vi "Position FLight Mode Enum.vi"(8 "error in (no error)":errorcluster, 10 "TabCtl Refnum":refnum<vi>, 11 "Enum Refnum":refnum<vi>) -> (0 "error out":errorcluster)   [LabVIEW 2014]
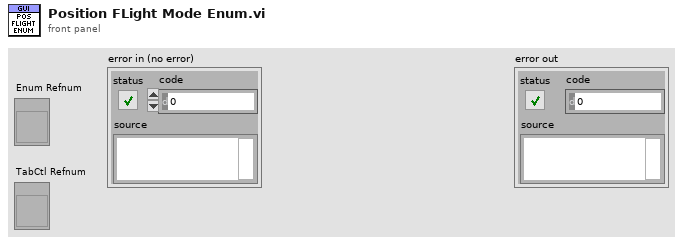
[diagram p1: front panel]
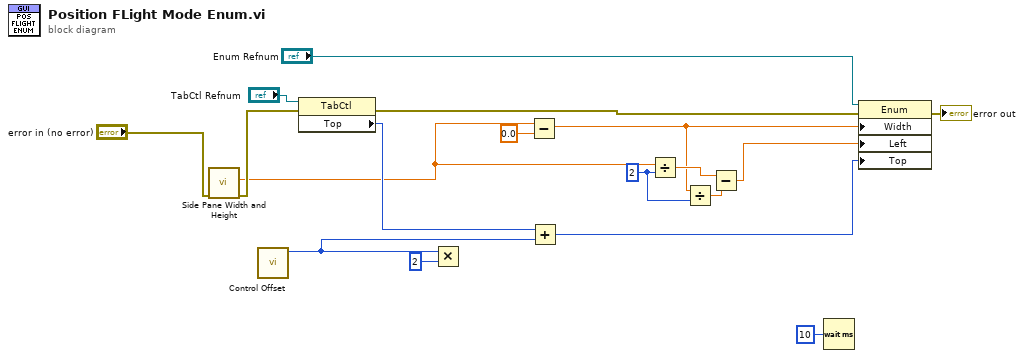
[diagram p0: block diagram]
diagram:
  w10 = u32 2 ("y")
  n1 = call "Side Pane Width and Height.vi"("error in (no error)"="error in (no error)") -> ("error out"=w3:errorcluster, "Width"=w2:dbl)  [unwired: 8 in, 1 out]
  n2 = call "Control Offset.vi"() -> ("Offset From Tab Edge in (px)"=w13:i32)  [unwired: 11 in]
  n3 = property class="TabCtl"(reference="TabCtl Refnum", error in=w3) -> (error out=w15:errorcluster, "Top"=w14:i32)  [unwired: 1 out]
  n4 = Multiply(x=w13, y=2) -> ()  [unwired: 1 out]
  n5 = Subtract(x=w2, y=0.0) -> (x-y=w9:dbl)
  n6 = Add(x=w14, y=w13) -> (x+y=w12:i32)
  n7 = Divide(x=w2, y=w10) -> (x/y=w11:dbl)
  n8 = Divide(x=w9, y=w10) -> (x/y=w8:dbl)
  n9 = Subtract(x=w11, y=w8) -> (x-y=w7:dbl)
  n10 = Wait (ms)(milliseconds to wait=u32 10) -> ()  [unwired: 1 out]
  n11 = property class="Enum"(reference="Enum Refnum", error in=w15, "Width"=w9, "Left"=w7, "Top"=w12) -> (error out=→"error out":errorcluster)  [unwired: 1 out]
